vi "niRFUtil FTW Get Window Bandwidths (bins).vi"(0 "FFT Window":T2=enum."Flat Top", 5 "Input Bandwidth Definition":T1=enum."Bin Width", 7 "Input Bandwidth (Hz)":dbl) -> (4 "Binwidth (Hz)":dbl, 6 "Bins (6dB)":dbl, 8 "Bins (3dB)":dbl)   [LabVIEW 2015, in "niRFUtil.lvlib"]
uses:
  niRFUtil.lvlib
  Includes/niRFUtil INC FFT Window.ctl
  Includes/niRFUtil INC Bandwidth Definition.ctl
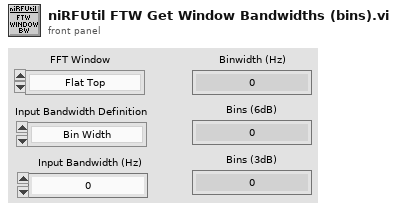
[diagram p1: front panel]
types:
  T1 = typedef "niRFUtil.lvlib/niRFUtil INC Bandwidth Definition.ctl" = enum16{"3dB", "6dB", "Bin Width", "ENBW"}
  T2 = typedef "niRFUtil.lvlib/niRFUtil INC FFT Window.ctl" = enum16{"None", "Flat Top", "Hanning", "Hamming", "Gaussian", "Blackman", "Blackman-Harris", "Kaiser-Bessel 70 dB", "Kaiser-Bessel 90 dB", "Kaiser-Bessel 110 dB"}
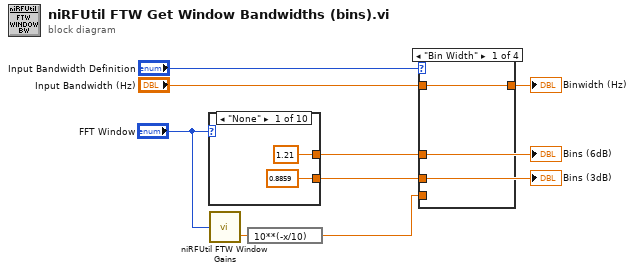
[diagram p0: block diagram]
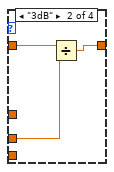
[diagram p2: hidden frame]
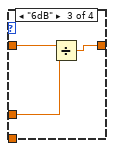
[diagram p3: hidden frame]
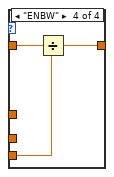
[diagram p4: hidden frame]
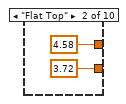
[diagram p5: hidden frame]
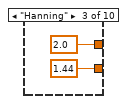
[diagram p6: hidden frame]
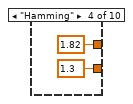
[diagram p7: hidden frame]
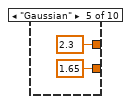
[diagram p8: hidden frame]
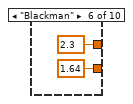
[diagram p9: hidden frame]
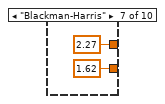
[diagram p10: hidden frame]
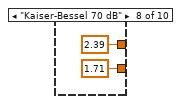
[diagram p11: hidden frame]
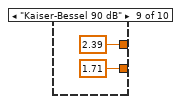
[diagram p12: hidden frame]
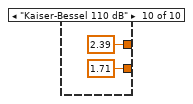
[diagram p13: hidden frame]
diagram:
  n1 = case shown="\"None\"" "FFT Window" {
    tunnel: [1.21 4.58 2.0 1.82 2.3 2.3 2.27 2.39 2.39 2.39] -> w5
    tunnel: [0.8859 3.72 1.44 1.3 1.65 1.64 1.62 1.71 1.71 1.71] -> w4
    frame "None" {
    }
    frame "Flat Top" {
    }
    frame "Hanning" {
    }
    frame "Hamming" {
    }
    frame "Gaussian" {
    }
    frame "Blackman" {
    }
    frame "Blackman-Harris" {
    }
    frame "Kaiser-Bessel 70 dB" {
    }
    frame "Kaiser-Bessel 90 dB" {
    }
    frame "Kaiser-Bessel 110 dB" {
    }
  }
  "Bins (6dB)" <- w5
  "Bins (3dB)" <- w4
  n2 = call "niRFUtil FTW Window Gains.vi"("Window"="FFT Window") -> ("-ENBW (dB-Hz)"=w3:sgl)  [unwired: 2 in, 1 out]
  n3 = expression code="10**(-x/10)"(w3) -> (w1:sgl)
  n4 = case shown="\"Bin Width\"" "Input Bandwidth Definition" {
    tunnel: [w29 w30 w34 w36] -> w7
    tunnel: "Input Bandwidth (Hz)" -> [w29 w32 w35 w38]
    tunnel: w5 -> [_ _ w33 _]
    tunnel: w4 -> [_ w31 _ _]
    tunnel: w1 -> [_ _ _ w37]
    frame "Bin Width" {
    }
    frame "3dB" {
      n5 = Divide(x=w32, y=w31) -> (x/y=w30:dbl)
    }
    frame "6dB" {
      n6 = Divide(x=w35, y=w33) -> (x/y=w34:dbl)
    }
    frame "ENBW" {
      n7 = Divide(x=w38, y=w37) -> (x/y=w36:dbl)
    }
  }
  "Binwidth (Hz)" <- w7
